vi "0xE8_Read_description_one_int_parameter.vi"(8 "error in":errorcluster, 10 "NumberIntParam":i32 format="%0d", 11 "paramUnicornIn in":T2) -> (0 "error out":errorcluster, 1 "Param":T1, 2 "Тип/версия устройства":string, 3 "paramUnicornIn out 2":T2)   [LabVIEW 2017, in "LV_Unicorn.lvlib"]
uses:
  LV_Unicorn.lvlib
  Control/unicorn_Param.ctl
  Control/unicorn_conn.ctl
  Control/unicorn_JSON.ctl
  Control/unicorn_ParamInt.ctl
  Control/unicorn_Telemetry.ctl
  Control/unicorn_Table.ctl
  Control/unicorn_ParamFloat.ctl
  Control/unicorn_DescriptParam.ctl
panel:
  out "Ответ":string
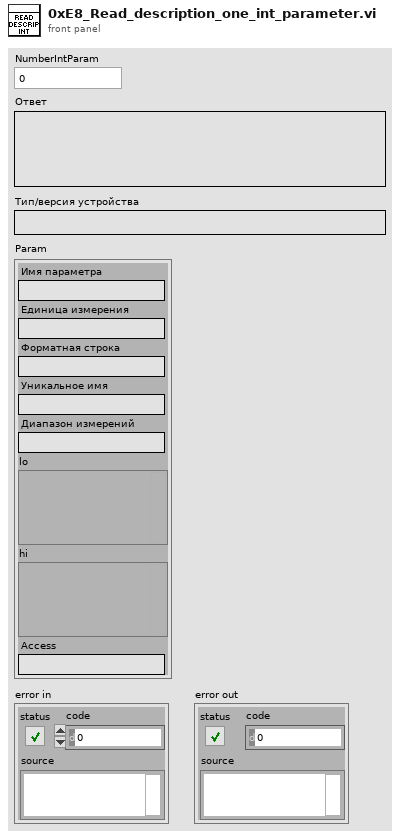
[diagram p1: front panel]
types:
  T1 = typedef "unicorn_DescriptParam.ctl" = cluster{"Имя параметра":string, "Единица измерения":string, "Форматная строка ":string, "Уникальное имя":string, "Диапазон измерений":string, "lo":variant, "hi":variant, "Access":string}
  T2 = typedef "LV_Unicorn.lvlib/unicorn_Param.ctl" = cluster{"conParam":T3, "Param":T4}
  T3 = typedef "LV_Unicorn.lvlib/unicorn_conn.ctl" = cluster{"ReadIntParam":bool, "ReadDescrParam":bool, "ReadFloatParam":bool, "debug":bool, "ReadJSON":bool, "IP_address":string, "N_attempts":i32, "type_con":enum16{"Serial", "TCP"}, "MB_address":i32, "VISA":refnum<visa-resource-name>, "connection ID":refnum<k5>, "nameDevices":string, "timeout":i32, "port":u16, "type_version":string, "baud_rate":u32, "VersionControl":bool, "TCP_conn":bool, "WindowSize":i32}
  T4 = typedef "LV_Unicorn.lvlib/unicorn_JSON.ctl" = cluster{"NumParam":cluster{"NTelem":i32, "NInt":i32, "NFloat":i32, "NTable":i32}, "ParamInt":T5, "Telemetry":T6, "Table":T7, "ParamFloat":T8}
  T5 = typedef "LV_Unicorn.lvlib/unicorn_ParamInt.ctl" = cluster{"ID":string, "Num":i32, "Name":string, "Type":string, "Enum":string, "Desc":string, "Unit":string, "Access":string, "FormatStr":string, "Min":i32, "Max":i32}[]
  T6 = typedef "LV_Unicorn.lvlib/unicorn_Telemetry.ctl" = cluster{"ID":string, "Num":i32, "Name":string, "Desc":string, "Unit":string, "FormatStr":string, "Min":i32, "Max":i32}[]
  T7 = typedef "LV_Unicorn.lvlib/unicorn_Table.ctl" = cluster{"Num":i32, "Access":string, "ColumnCount":i32, "NeedParamPrepare":bool, "Columns":cluster{"Column":i32, "Desc":string, "Name":string}[], "DataType":string, "FormatStr":string, "ID":string, "Name":string, "RowCount":i32, "Rows":cluster{"Desc":string, "ID":string, "Max":i32, "Min":i32, "Name":string, "Row":i32, "Unit":string}[], "Type":string}[]
  T8 = typedef "LV_Unicorn.lvlib/unicorn_ParamFloat.ctl" = cluster{"ID":string, "Num":i32, "Name":string, "Type":string, "Enum":string, "Desc":string, "Unit":string, "Access":string, "FormatStr":string, "Min":sgl, "Max":sgl}[]
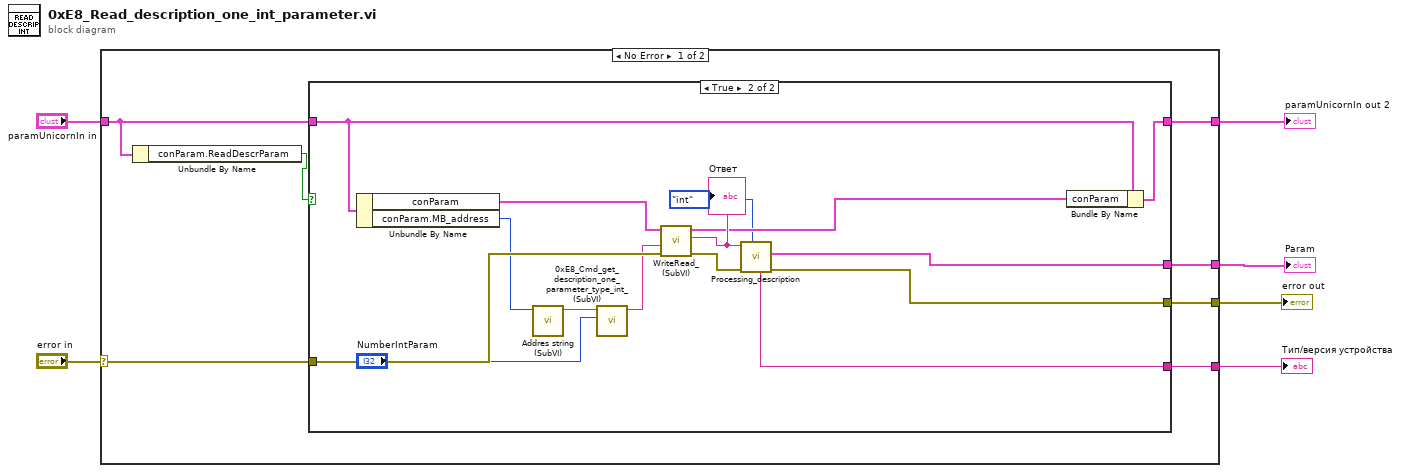
[diagram p0: block diagram]
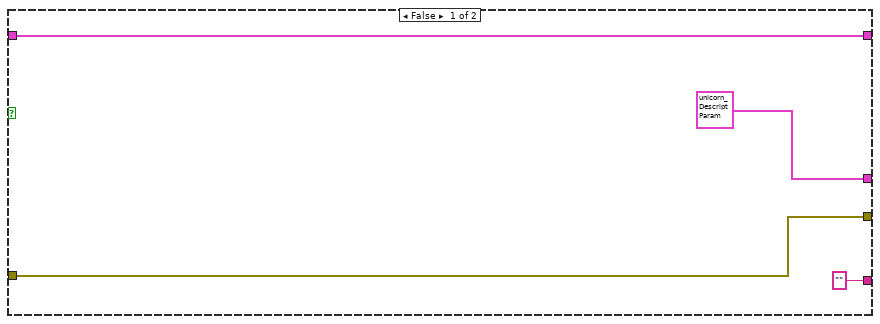
[diagram p2: hidden frame]
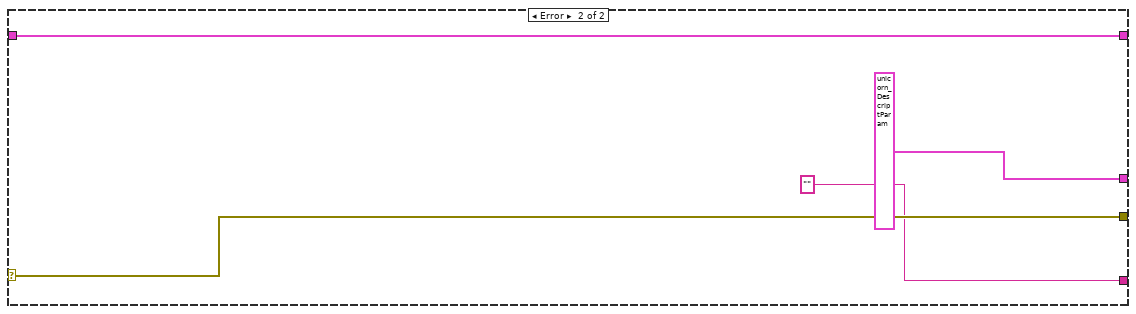
[diagram p3: hidden frame]
diagram:
  n1 = case shown="No Error" "error in" {
    selector: "error in" -> [w13 w36]
    tunnel: [w12 w36] -> w6
    tunnel: "paramUnicornIn in" -> [w8 w35]
    tunnel: [w9 w35] -> w4
    tunnel: [w11 T1 {"Имя параметра"="", "Единица измерения"="", "Форматная строка "="", "Уникальное имя"="", "Диапазон измерений"="", "lo"=variant, "hi"=variant, "Access"=""} ("Param")] -> w2
    tunnel: [w10 "" ("Ответ")] -> w1
    frame No Error {
      n2 = Unbundle By Name(w8) -> ("conParam.ReadDescrParam"=w7:bool)
      n3 = case shown="True" w7 {
        tunnel: w13 -> [w15 w31]
        tunnel: [w15 w28] -> w12
        tunnel: [T1 {"Имя параметра"="", "Единица измерения"="", "Форматная строка "="", "Уникальное имя"="", "Диапазон измерений"="", "lo"=variant, "hi"=variant, "Access"=""} ("Param") w27] -> w11
        tunnel: ["" ("Тип/версия устройства") w26] -> w10
        tunnel: [w17 w25] -> w9
        tunnel: w8 -> [w17 w23]
        frame False {
        }
        frame True {
          n4 = Unbundle By Name(w23) -> ("conParam"=w32:T3, "conParam.MB_address"=w22:i32)
          n5 = call "Addres string (SubVI).vi"("Адрес"=w22) -> ("String"=w21:string)  [unwired: 10 in]
          n6 = call "0xE8_Cmd_get_description_one_parameter_type_int_(SubVI).vi"("NumberIntParam"="NumberIntParam", "String in"=w21) -> ("String out"=w20:string)  [unwired: 9 in]
          n7 = call "WriteRead_(SubVI).vi"("error in"=w31, "Запрос"=w20, "ParamIn"=w32) -> ("error out"=w30:errorcluster, "Ответ"=w29:string, "ParamOut"=w24:T3)  [unwired: 4 in, 2 out]
          "Ответ" <- w29
          n8 = call "Processing_description.vi"("type"=enum16{"int", "float"}."int", "error in"=w30, "Ответ устройства"=w29) -> ("error out"=w28:errorcluster, "Param"=w27:T1, "Тип/версия устройства"=w26:string)  [unwired: 5 in, 1 out]
          n9 = Bundle By Name(cluster=w23, "conParam"=w24) -> (w25:T2)
        }
      }
    }
    frame Error {
    }
  }
  "error out" <- w6
  "paramUnicornIn out 2" <- w4
  "Param" <- w2
  "Тип/версия устройства" <- w1
